vi "CALC_MARK_FUNC_TRAC_ON_OFF.vi"(0 "VISA IN":refnum<visa-resource-name>, 1 "Marker number":i32=1, 2 "Track ON/OFF":bool, 5 "error in":errorcluster, 7 "Channel":i32=1) -> (14 "VISA Out":refnum<visa-resource-name>, 19 "error out":errorcluster)   [LabVIEW 2018, in "PNA-X.lvlib"]
doc: "CALCulate<cnum>:MARKer<mkr>:FUNCtion:TRACking <ON | OFF> \n(Read-Write) Sets the tracking capability for the specified marker. The tracking function finds the \nselected search function every sweep. In effect, turning Tracking ON is the same as doing a \nCALC:MARK:FUNC:EXECute command every sweep. \nSee Critical Note \nParameters \n<cnum> Channel number of the measurement. There must be a selected measurement \non that channel. If unspecified, <cnum> is set to 1. \n<mkr> Any marker number from 1 to 10; if unspecified, value is set to 1. \n<ON | OFF> ON (or 1) - The specified marker will \"Track\" (find) the selected function \nevery sweep. \nOFF (or 0) - The specified marker will find the selected function only when \nthe CALC:MARK:FUNC:EXECute command is sent. \nExamples CALC:MARK:FUNC:TRAC ON \ncalculate2:marker8:function:tracking off \nQuery Syntax CALCulate<cnum>:MARKer<mkr>:FUNCtion:TRACking? \n1538\n\nReturn Type Boolean (1 = ON, 0 = OFF) \nDefault OFF"
uses:
  PNA-X.lvlib
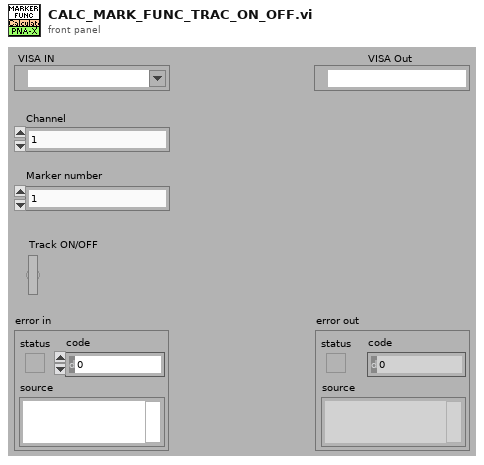
[diagram p1: front panel]
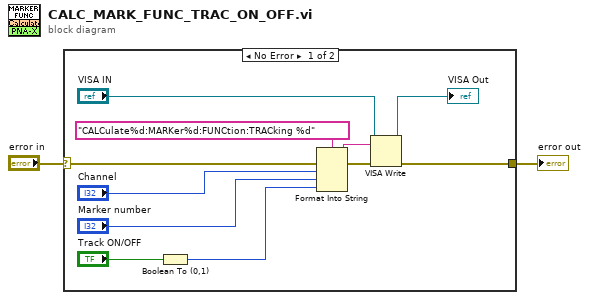
[diagram p0: block diagram]
diagram:
  n1 = case shown="No Error" "error in" {
    selector: "error in" -> [w13 w14]
    tunnel: [w8 w14] -> w1
    frame No Error {
      n2 = Boolean To (0,1)(Boolean="Track ON/OFF") -> (0, 1=w3:i16)
      n3 = Format Into String(format string="CALCulate%d:MARKer%d:FUNCtion:TRACking %d" ("Cmdline"), error in=w13, "Channel", "Marker number", w3) -> (resulting string=w11:string, error out=w12:errorcluster)  [unwired: 1 in]
      n4 = VISA Write(VISA resource name="VISA IN", write buffer=w11, error in (no error)=w12) -> (VISA resource name out=→"VISA Out":refnum<visa-resource-name>, error out=w8:errorcluster)  [unwired: 1 out]
    }
    frame Error {
    }
  }
  "error out" <- w1
